vi "StoreManipulator.vi"(8 "error in (no error)":errorcluster, 11 "Elevator Concrete in":refnum<class "Elevator Concrete.lvclass">) -> (0 "error out":errorcluster, 3 "Elevator Concrete out":refnum<class "Elevator Concrete.lvclass">)   [LabVIEW 2018, in "Elevator.lvlib" / "Elevator Concrete.lvclass"]
uses:
  Elevator Concrete.lvclass
  Controls/Elevator Position.ctl
  Elevator.lvclass
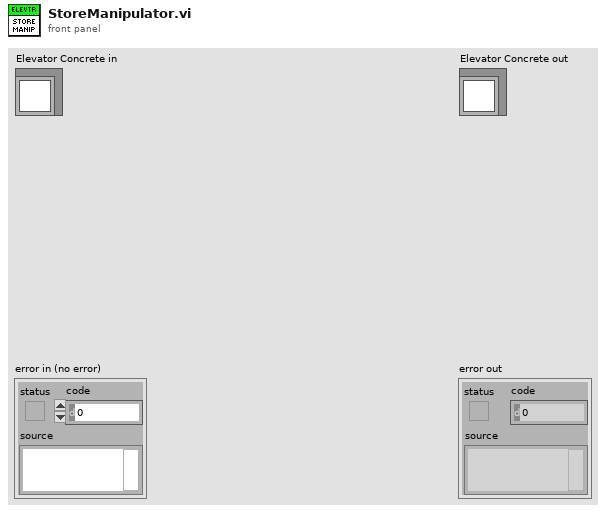
[diagram p1: front panel]
types:
  T1 = typedef "Elevator.lvlib/Elevator.lvclass/Elevator Position.ctl" = enum16{"C0, Cargo Ground", "C1, LV1 Cargo", "C2, Cargo Ship Cargo", "H0, LV1 Hatch", "H1, LV2 Hatch"}
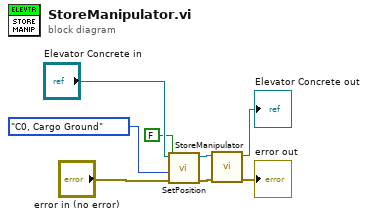
[diagram p0: block diagram]
diagram:
  n1 = call-dynamic "SetPosition.vi"("error in (no error)"="error in (no error)", "Position"=Elevator_Position."C0, Cargo Ground", "Hach Grabed?"=FALSE, "Elevator Concrete in"="Elevator Concrete in") -> ("error out"=w6:errorcluster, "Elevator Concrete out"=w4:refnum<class "Elevator Concrete.lvclass">)  [unwired: 6 in]
  n2 = call-parent "StoreManipulator.vi"("error in (no error)"=w6, "Elevator in"=w4) -> ("error out"=→"error out":errorcluster, "Elevator out"=→"Elevator Concrete out":refnum<class "Elevator Concrete.lvclass">)  [unwired: 8 in]
